vi "2angleServo-WorkOnMouse.vi"() -> ()   [LabVIEW 2019]
uses:
  <vilib>/LabVIEW Interface for Arduino/Type Defs/Board Type.ctl
  <vilib>/Utility/inputDevices.llb/mouseAcquire.vi
  <vilib>/Utility/inputDevices.llb/closeMouse.vi
  <vilib>/LabVIEW Interface for Arduino/LabVIEW Interface for Arduino.lvlib
panel:
  out "horizontal":u8
  out "vertical":u8
  in  "div vertic":dbl=2.0
  in  "div horiz":dbl=2.0
  out "button 1":bool
  out "Waveform Chart":T1(graph)
  out "err mouse":errorcluster
  out "err arduino":errorcluster
  in  "stop":bool
  in  "VISA resource":refnum<visa-resource-name>
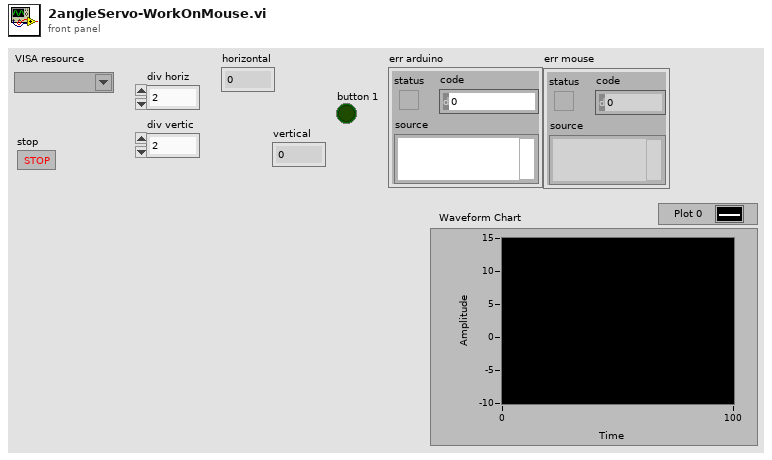
[diagram p1: front panel]
types:
  T1 = cluster{"Horizontal":i32, "Vertical":i32, "Scrolling":i32}
  T2 = typedef "LabVIEW Interface for Arduino.lvlib/Board Type.ctl" = enum16{"Uno", "Dimuelanove w/Atmega 328", "Mega 2560"}
  T3 = typedef "LabVIEW Interface for Arduino.lvlib/Arduino Resource.ctl" = cluster{"VISA resource":refnum<visa-resource-name>, "Board Type":T2, "Connection Type":enum8{"USB / Serial"}, "Bytes Per Packet (15)":u8}
  T4 = cluster{"button 1":bool, "button 2":bool, "button 3":bool, "button 4":bool}
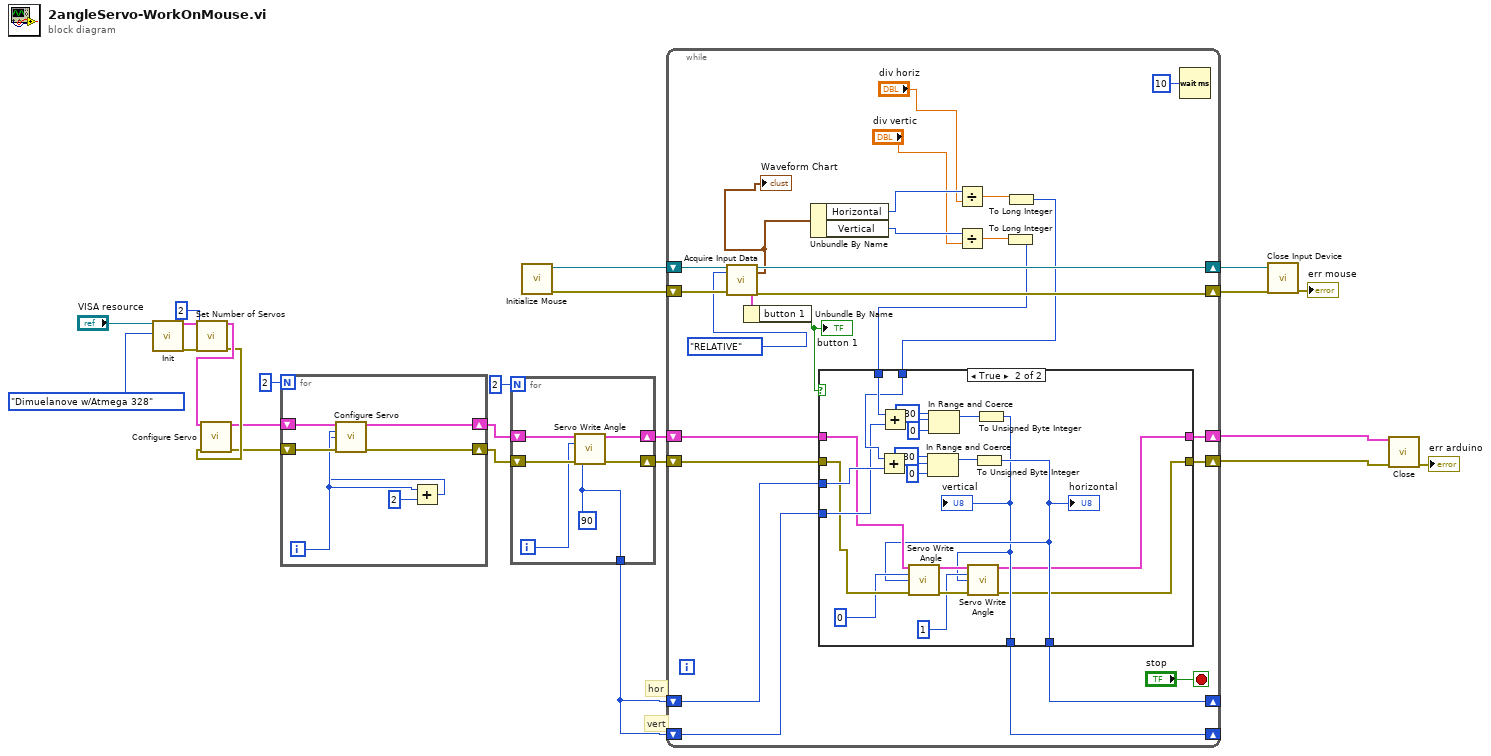
[diagram p0: block diagram]
diagram:
  # "vert"
  # "hor"
  n1 = call <vilib>:"Init.vi"("VISA resource"="VISA resource", "Board Type (Uno)"=Board_Type."Dimuelanove w/Atmega 328") -> ("Arduino Resource"=w22:T3, "error out"=w21:errorcluster)  [unwired: 16 in]
  n2 = call <vilib>:"Set Number of Servos.vi"("Arduino Resource"=w22, "Number Of Servos (1)"=u8 2, "error in"=w21) -> ("Arduino Resource"=w19:T3, "error out"=w18:errorcluster)  [unwired: 11 in]
  n3 = call <vilib>:"Configure Servo.vi"("Arduino Resource"=w19, "error in"=w18) -> ("Arduino Resource"=w17:T3, "error out"=w16:errorcluster)  [unwired: 12 in]
  n4 = for {
    N: 2 -> [_]
    shift-right: [w26] -> w14
    shift-left: w17 -> [w31]
    shift-right: [w25] -> w13
    shift-left: w16 -> [w30]
    i -> [w29]
    n5 = Add(x=w29, y=2) -> (x+y=w27:i32)
    n6 = call <vilib>:"Configure Servo.vi"("Arduino Resource"=w31, "Servo Number (0)"=w29, "DIO Pin (2)"=w27, "error in"=w30) -> ("Arduino Resource"=w26:T3, "error out"=w25:errorcluster)  [unwired: 10 in]
  }
  n7 = for {
    N: 2 -> [_]
    shift-right: [w35] -> w12
    shift-left: w14 -> [w37]
    shift-right: [w34] -> w11
    shift-left: w13 -> [w36]
    tunnel: [w32] -> w6
    i -> [w33]
    w32 = u8 90 ("Angle (Degrees)")
    n8 = call <vilib>:"Servo Write Angle.vi"("Arduino Resource"=w37, "Servo Number"=w33, "Angle (Degrees)"=w32, "error in"=w36) -> ("Arduino Resource"=w35:T3, "error out"=w34:errorcluster)  [unwired: 10 in]
  }
  n9 = call <vilib>:"Initialize Mouse.vi"() -> ("error out"=w4:errorcluster, "device ID"=w5:refnum<k1>)  [unwired: 10 in]
  n10 = while {
    shift-right: [w47] -> w9
    shift-left: w12 -> [w46]
    shift-right: [w45] -> w8
    shift-left: w11 -> [w44]
    shift-right: [w38] -> _
    shift-left: w6 -> [w41]
    shift-right: [w39] -> _
    shift-left: w6 -> [w40]
    shift-right: [w59] -> w3
    shift-left: w5 -> [w61]
    shift-right: [w58] -> w2
    shift-left: w4 -> [w60]
    stop <- "stop" stop-if-true
    n11 = call-poly <vilib>:"Acquire Input Data.vi"("device ID"=w61, "key mode"=enum16{"RELATIVE", "ABSOLUTE"}."RELATIVE", "error in (no error)"=w60) -> ("device ID"=w59:refnum<k1>, "axis info"=w55:T1, "button info"=w56:T4, "error out"=w58:errorcluster)  [unwired: 13 in]
    "Waveform Chart" <- w55
    n12 = Unbundle By Name(w56) -> ("button 1"=w48:bool)
    "button 1" <- w48
    n13 = Unbundle By Name(w55) -> ("Horizontal"=w54:i32, "Vertical"=w52:i32)
    n14 = Divide(x=w54, y="div horiz") -> (x/y=w49:dbl)
    n15 = Divide(x=w52, y="div vertic") -> (x/y=w50:dbl)
    n16 = To Long Integer(number=w50) -> (32bit integer=w43:i32)
    n17 = To Long Integer(number=w49) -> (32bit integer=w42:i32)
    n18 = case shown="True" w48 {
      tunnel: [w67 w69] -> w47
      tunnel: w46 -> [w67 w77]
      tunnel: [w66 w68] -> w45
      tunnel: w44 -> [w66 w76]
      tunnel: w43 -> [w65 w89]
      tunnel: w42 -> [w64 w88]
      tunnel: w41 -> [_ w87]
      tunnel: w40 -> [_ w86]
      tunnel: [w65 w70] -> w39
      tunnel: [w64 w71] -> w38
      frame False {
      }
      frame True {
        n19 = Add(x=w88, y=w87) -> (x+y=w84:i32)
        n20 = Add(x=w89, y=w86) -> (x+y=w85:i32)
        n21 = In Range and Coerce(upper limit=180, x=w84, lower limit=0) -> (coerced(x)=w78:i32)  [unwired: 1 out]
        n22 = In Range and Coerce(upper limit=180, x=w85, lower limit=0) -> (coerced(x)=w79:i32)  [unwired: 1 out]
        n23 = To Unsigned Byte Integer(number=w78) -> (unsigned 8bit integer=w71:u8)
        "horizontal" <- w71
        n24 = call <vilib>:"Servo Write Angle.vi"("Arduino Resource"=w77, "Servo Number"=u8 0, "Angle (Degrees)"=w71, "error in"=w76) -> ("Arduino Resource"=w75:T3, "error out"=w74:errorcluster)  [unwired: 10 in]
        n25 = To Unsigned Byte Integer(number=w79) -> (unsigned 8bit integer=w70:u8)
        "vertical" <- w70
        n26 = call <vilib>:"Servo Write Angle.vi"("Arduino Resource"=w75, "Servo Number"=u8 1, "Angle (Degrees)"=w70, "error in"=w74) -> ("Arduino Resource"=w69:T3, "error out"=w68:errorcluster)  [unwired: 10 in]
      }
    }
    n27 = Wait (ms)(milliseconds to wait=u32 10) -> ()  [unwired: 1 out]
  }
  n28 = call-poly <vilib>:"Close Input Device.vi"("error in (no error)"=w2, "device ID"=w3) -> ("error out"=→"err mouse":errorcluster)  [unwired: 8 in]
  n29 = call <vilib>:"Close.vi"("Arduino Resource"=w9, "error in"=w8) -> ("error out"=→"err arduino":errorcluster)  [unwired: 13 in]
